vi "指示灯闪烁.vi"() -> ()   [LabVIEW 2015]
panel:
  out "布尔":bool
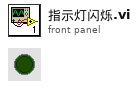
[diagram p1: front panel]
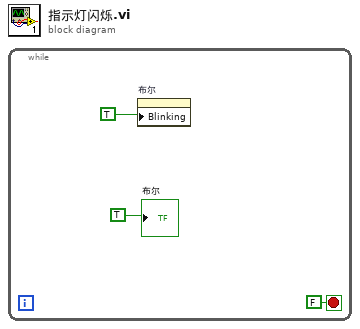
[diagram p0: block diagram]
diagram:
  n1 = while {
    stop <- FALSE stop-if-true
    n2 = property on="布尔" class="Bool (严格)"("Blinking"=TRUE) -> ()  [unwired: 2 in, 2 out]
    "布尔" <- TRUE
  }
